vi "TestHysteresis.vi"() -> ()   [LabVIEW 2022 SP3]
panel:
  in  "stop":bool
  in  "Input":dbl format="%.2p"
  in  "type":enum16{"Percentage", "level"}(ring)
  out "ACT_Dv_too_large":bool
  out "error out":errorcluster
  in  "error in (no error)":errorcluster
  in  "level":dbl format="%.2p"
  in  "hysteresis":dbl=0.3 format="%#_13g"
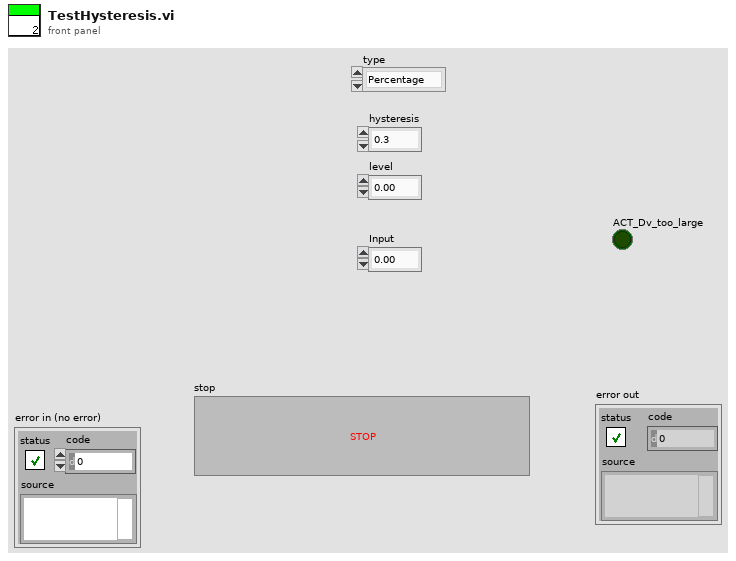
[diagram p1: front panel]
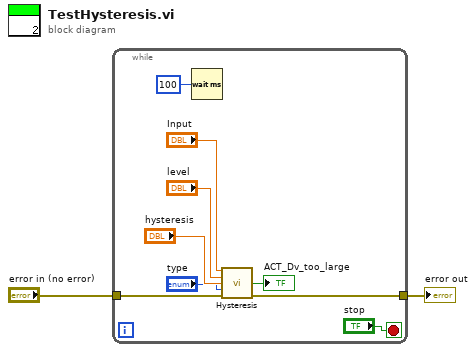
[diagram p0: block diagram]
diagram:
  n1 = while {
    tunnel: [w8] -> w2
    tunnel: "error in (no error)" -> [w7]
    stop <- "stop" stop-if-true
    n2 = Wait (ms)(milliseconds to wait=u32 100) -> ()  [unwired: 1 out]
    n3 = call "Hysteresis.vi"("Input"="Input", "level"="level", "hysteresis"="hysteresis", "type"="type", "error in (no error)"=w7) -> ("ACT_Dv_too_large"=→"ACT_Dv_too_large":bool, "error out"=w8:errorcluster)  [unwired: 9 in]
  }
  "error out" <- w2
